vi "SaveNAFile.vi"(0 "delimiter (\\t)":string="\t", 4 "format (%.3f)":string="%.3f", 5 "append to file? (new file:F)":bool, 7 "XY":cluster{dbl[], dbl[]}(graph), 8 "file path (dialog if empty)":path) -> (3 "new file path (Not A Path if cancelled)":path)   [LabVIEW 2013]
doc: "Converts a 2D or 1D array of strings, signed integers, or double-precision numbers to a text string and writes the string to a new byte stream file or appends the string to an existing file. Wire data to the <B>2D data</B> input or <B>1D data</B> input to determine the polymorphic instance to use or manually select the instance.\n\nUse this VI to transpose or separate data.\n\n<B>Note</B> To format with Microsoft Excel, use ActiveX with LabVIEW or the Report Generation Toolkit for Microsoft Office."
uses:
  <vilib>/Utility/error.llb/DialogType.ctl
panel:
  in  "prompt":string="Choose file to write."
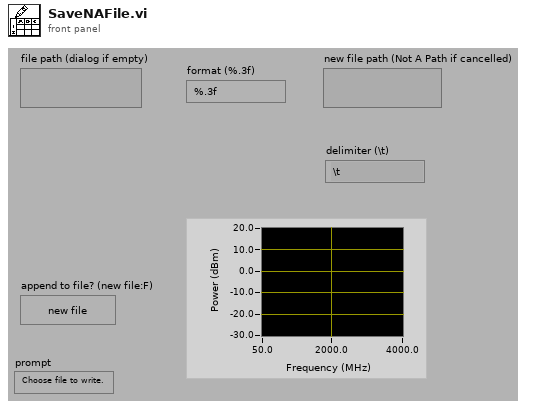
[diagram p1: front panel]
types:
  T1 = typedef "DialogType.ctl" = u16
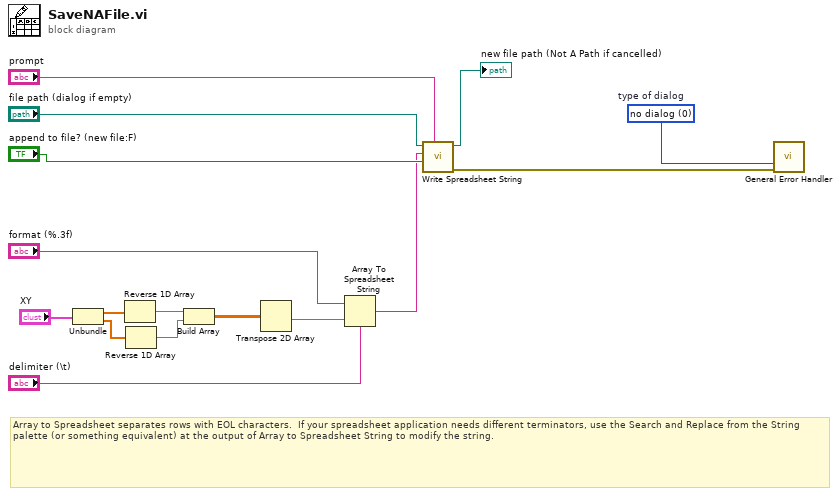
[diagram p0: block diagram]
diagram:
  w7 = T1 0 items=["no dialog", "OK message", "continue or stop message", "OK message + warnings", "continue/stop + warnings"]  # type of dialog
  # "Array to Spreadsheet separates rows with EOL characters.  If your spreadsheet application needs different terminators, use the Search and Replace from the String palette (or something equivalent) at the output of Array to Spreadsheet String to modify the string."
  n1 = Unbundle("XY") -> (w6:dbl[], w4:dbl[])
  n2 = Reverse 1D Array(array=w6) -> (reversed array=w5:dbl[])
  n3 = Reverse 1D Array(array=w4) -> (reversed array=w3:dbl[])
  n4 = Build Array(w5, w3) -> (w1:dbl[][])
  n5 = Transpose 2D Array(2D array=w1) -> (transposed array=w14:dbl[][])
  n6 = Array To Spreadsheet String(delimiter (Tab)="delimiter (\\t)", array=w14, 3:"format (%.3f)") -> (spreadsheet string=w9:string)
  n7 = call <vilib>:"Write Spreadsheet String.vi"("prompt"="prompt", "append to file? (new file:F)"="append to file? (new file:F)", "spreadsheet string"=w9, "file path (dialog if empty)"="file path (dialog if empty)") -> ("error out"=w8:errorcluster, "path"=→"new file path (Not A Path if cancelled)":path)  [unwired: 6 in]
  n8 = call <vilib>:"General Error Handler.vi"("type of dialog (OK msg:1)"=w7, "error in (no error)"=w8) -> ()  [unwired: 9 in, 5 out]
